vi "Pressure Sensor (Set).vi"(6 "ISOBUS address":T4=-1 caption="ISOBUS address (-1)", 8 "error in":errorcluster, 10 "Sensor Type":T3, 11 "Mercury Reference In":T5) -> (0 "error out":errorcluster, 2 "Response":T1, 3 "Mercury Reference Out":T5, 4 "Valid?":T2)   [LabVIEW 2013, in "Mercury iXX.lvlib" / "Pressure.lvlib"]
doc: "Set the sensor type of the selected pressure device."
uses:
  Pressure.lvlib
  Mercury iXX.lvlib
  Private/Controls/Command Verbs.ctl
  Controls/Response String.ctl
  Controls/Is Valid LED.ctl
  Controls/Comms Transport Layer.ctl
  Controls/Mercury Reference.ctl
  Controls/Pressure Sensor Type.ctl
  Controls/ISOBus Address.ctl
  Private/Controls/Query Dynamic Reference.ctl
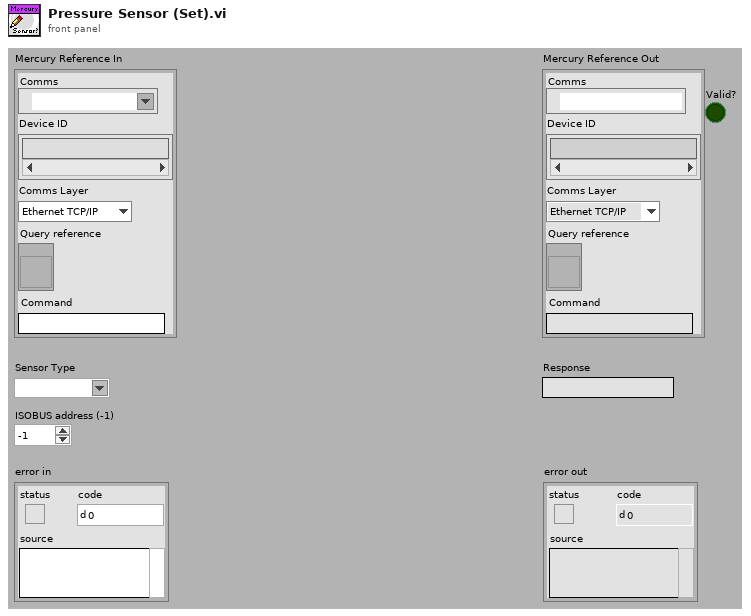
[diagram p1: front panel]
types:
  T1 = typedef "Mercury iXX.lvlib/Response String.ctl" = string
  T2 = typedef "Mercury iXX.lvlib/Is Valid LED.ctl" = bool
  T3 = typedef "Mercury iXX.lvlib/Pressure.lvlib/Pressure Sensor Type.ctl" = string
  T4 = typedef "Mercury iXX.lvlib/ISOBus Address.ctl" = i32
  T5 = typedef "Mercury iXX.lvlib/Mercury Reference.ctl" = cluster{"Comms":refnum<visa-resource-name>, "Device ID":string[], "Comms Layer":T6, "Command":string, "Query reference":T7}
  T6 = typedef "Mercury iXX.lvlib/Comms Transport Layer.ctl" = enum16{"Ethernet TCP/IP", "USB", "ISOBus - RS-232", "GPIB"}
  T7 = typedef "Mercury iXX.lvlib/Query Dynamic Reference.ctl" = refnum<vi>
  T8 = typedef "Mercury iXX.lvlib/Command Verbs.ctl" = string
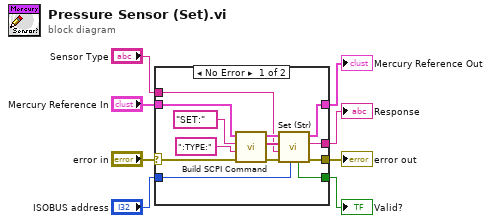
[diagram p0: block diagram]
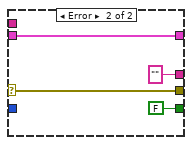
[diagram p2: hidden frame]
diagram:
  n1 = case shown="No Error" "error in" {
    selector: "error in" -> [w9 w22]
    tunnel: "Mercury Reference In" -> [w17 w25]
    tunnel: "Sensor Type" -> [w16 _]
    tunnel: [w14 w22] -> w6
    tunnel: "ISOBUS address" -> [w13 _]
    tunnel: [w12 T2 FALSE ("Valid?")] -> w4
    tunnel: [w11 T1 "" ("Response")] -> w3
    tunnel: [w10 w25] -> w2
    frame No Error {
      n2 = call "Build SCPI Command.vi"("error in"=w9, "Noun(s)"=":TYPE:" ("Command"), "Verb"=T8 "SET:", "Mercury Reference In"=w17) -> ("error out"=w18:errorcluster, "SCPI Message(s)"=w19:string[], "Mercury Reference Out"=w20:T5)  [unwired: 5 out]
      n3 = call "Set (Str).vi"("ISOBUS address"=w13, "error in"=w18, "Command Value (Str)"=w16, "SCPI Message(s)"=w19, "Mercury Reference In"=w20) -> ("error out"=w14:errorcluster, "Response"=w11:T1, "Mercury Reference Out"=w10:T5, "Valid?"=w12:T2)  [unwired: 3 out]
    }
    frame Error {
    }
  }
  "Mercury Reference Out" <- w2
  "error out" <- w6
  "Valid?" <- w4
  "Response" <- w3
